vi "(SubVI)_ UpdateImpTabParameters.vi"(1 "Stim Galvo Cluster":T2, 2 "Imp Tab Parameters":T1) -> (0 "Updated Parameters":T1)   [LabVIEW 2012]
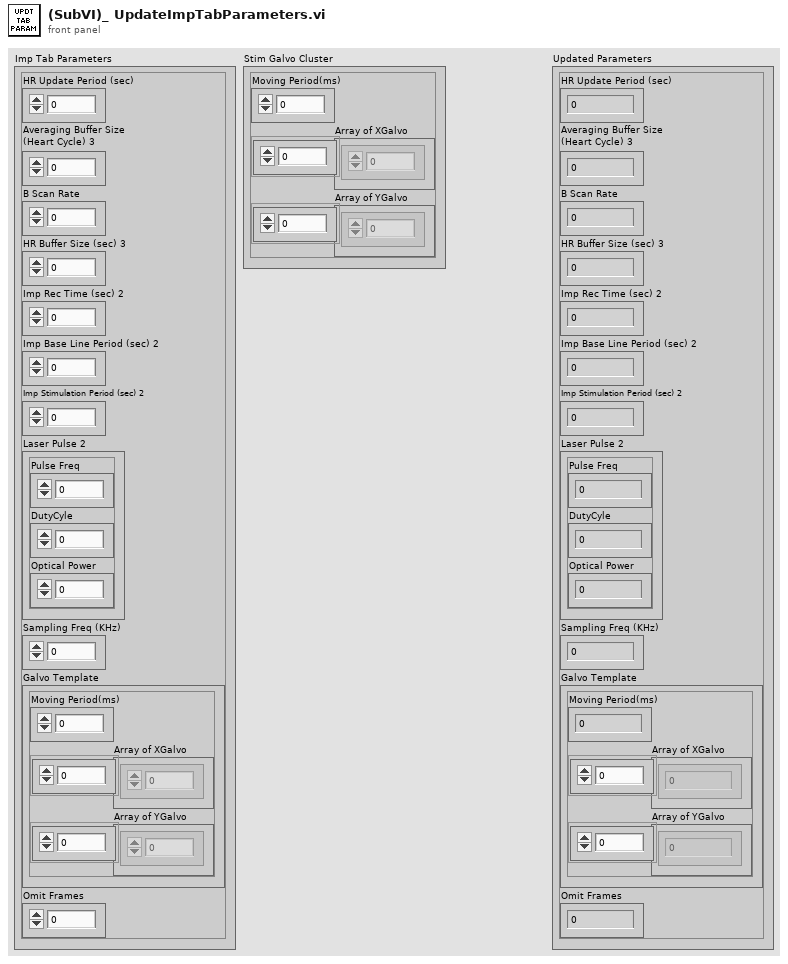
[diagram p1: front panel]
types:
  T1 = cluster{"HR Update Period (sec)":i32, "Averaging Buffer Size\n(Heart Cycle) 3":dbl, "B Scan Rate":dbl, "HR Buffer Size (sec) 3":dbl, "Imp Rec Time (sec) 2":dbl, "Imp Base Line Period (sec) 2":dbl, "Imp Stimulation Period (sec) 2":dbl, "Laser Pulse 2":cluster{"Pulse Freq":dbl, "DutyCyle":dbl, "Optical Power":dbl}, "Sampling Freq (KHz)":dbl, "Galvo Template":cluster{"Moving Period(ms)":dbl, "Array of XGalvo":dbl[], "Array of YGalvo":dbl[]}, "Omit Frames":i32}
  T2 = cluster{"Moving Period(ms)":dbl, "Array of XGalvo":dbl[], "Array of YGalvo":dbl[]}
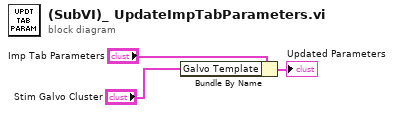
[diagram p0: block diagram]
diagram:
  n1 = Bundle By Name(cluster="Imp Tab Parameters", "Galvo Template"="Stim Galvo Cluster") -> (→"Updated Parameters":T1)
